vi "Run_Init Core.vi"(0 "functionbase in":refnum<class "functionbase.lvclass">, 11 "error in (no error)":errorcluster) -> (4 "functionbase out":refnum<class "functionbase.lvclass">, 15 "error out":errorcluster)   [LabVIEW 2019, in "LSL.lvlib" / "functionbase.lvclass"]
uses:
  functionbase.lvclass
  functionbase.lvclass/functionbase.ctl
  properties/Read Func Full String.vi
  properties/Read RT Variables.vi
  variables/RT Variables/RT Variables.lvclass
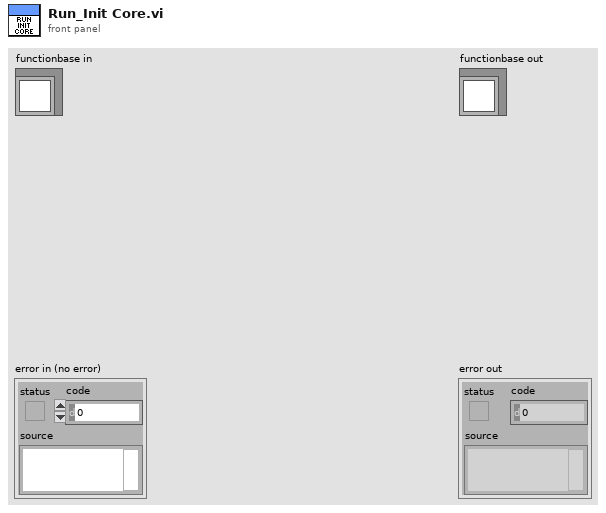
[diagram p1: front panel]
types:
  T1 = typedef "Datatype.ctl" = enum16{"Null", "Numeric", "String", "Bool", "Numeric 1D", "String 1D", "Bool 1D", "Numeric 2D", "String 2D", "Bool 2D", "Variant"}
  T2 = typedef "Valuetype.ctl" = enum16{"Value", "Variable", "Function"}
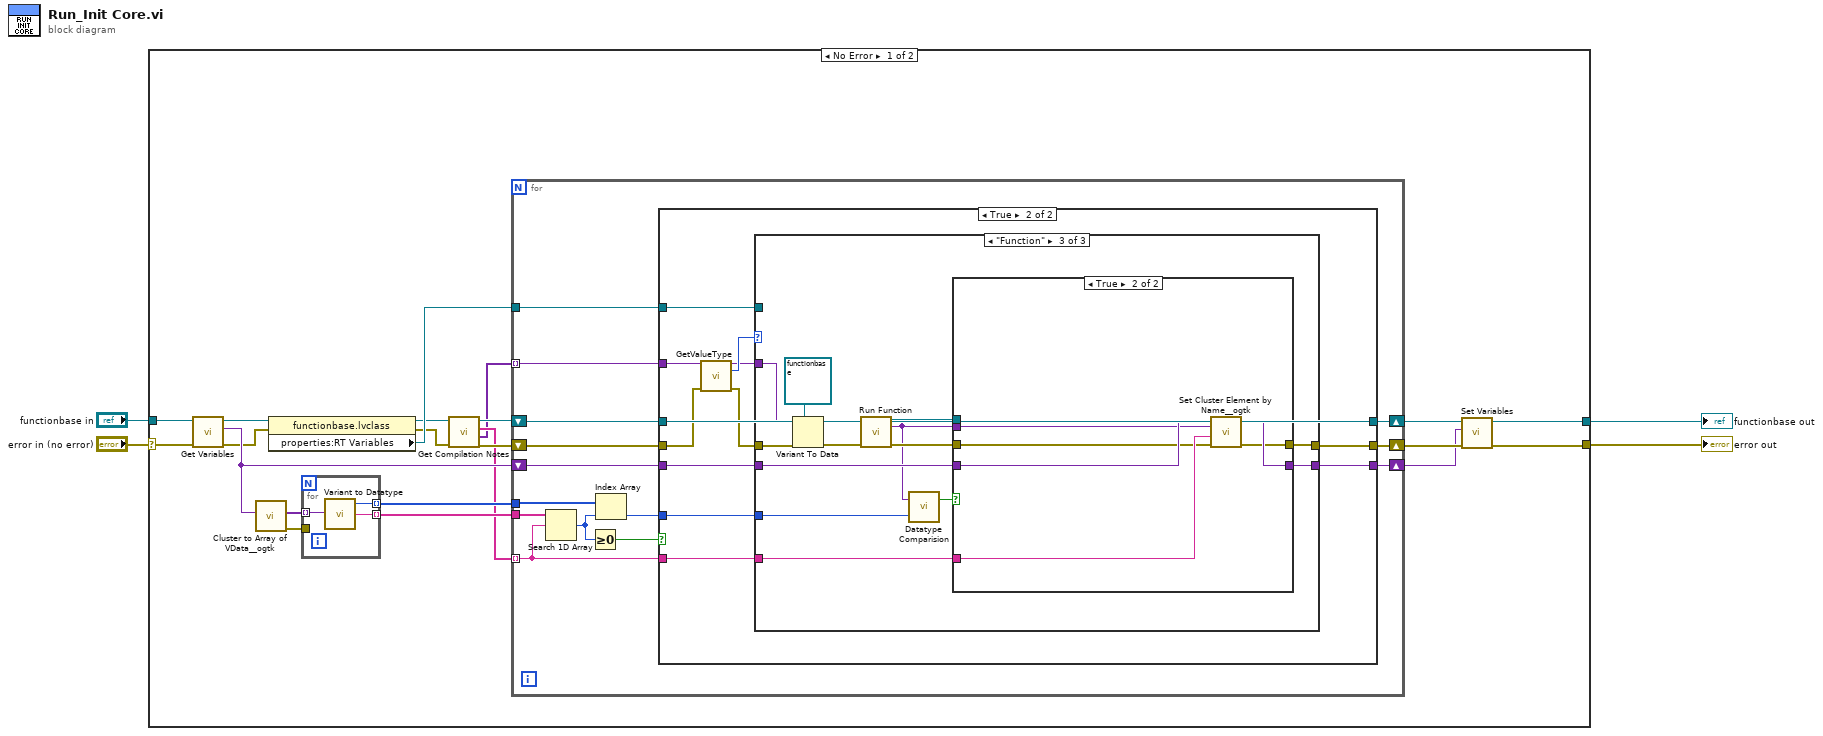
[diagram p0: block diagram]
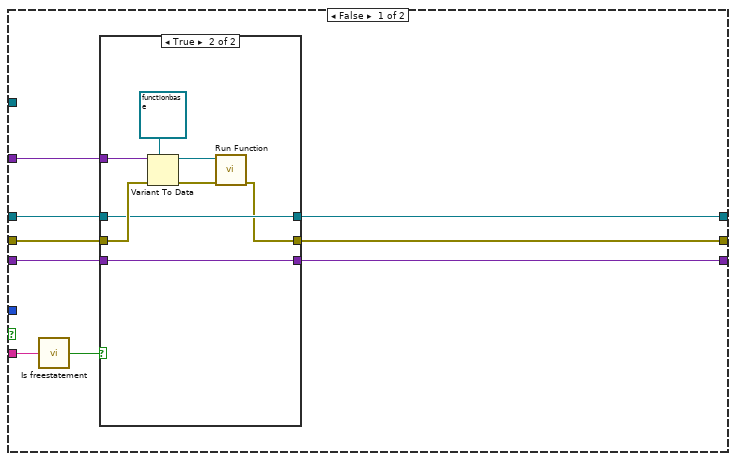
[diagram p2: hidden frame]
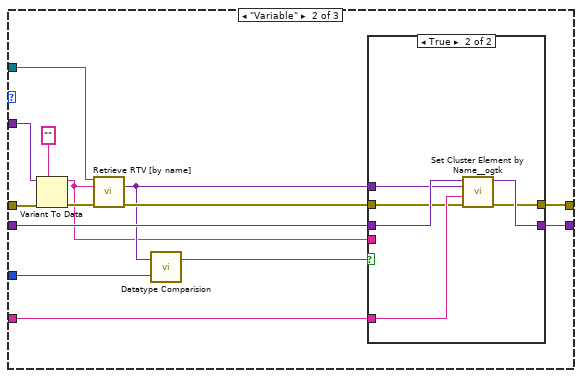
[diagram p5: hidden frame]
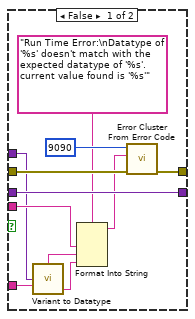
[diagram p6: hidden frame]
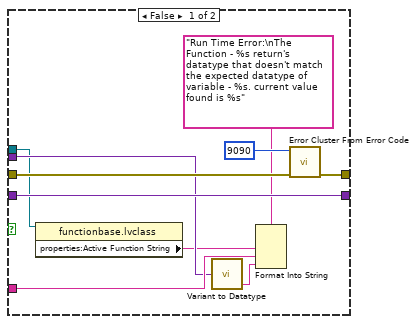
[diagram p7: hidden frame]
diagram:
  n1 = case shown="No Error" "error in (no error)" {
    selector: "error in (no error)" -> [w24 w138]
    tunnel: [w16 w138] -> w3
    tunnel: [w15 w137] -> w1
    tunnel: "functionbase in" -> [w23 w137]
    frame No Error {
      n2 = call-dynamic "Get Variables.vi"("error in (no error)"=w24, "functionbase in"=w23) -> ("error out"=w12:errorcluster, "Variables"=w20:variant, "functionbase out"=w13:refnum<class "functionbase.lvclass">)  [unwired: 7 in]
      n3 = call <userlib>:"Cluster to Array of VData__ogtk.vi"("Cluster"=w20) -> ("error out"=w22:errorcluster, "Array of VData"=w25:variant[])  [unwired: 9 in]
      n4 = property class="functionbase.lvclass"(reference=w13, error in=w12) -> (reference out=w10:refnum<class "functionbase.lvclass">, error out=w7:errorcluster, "properties:RT Variables"=w11:refnum<class "RT Variables.lvclass">)
      n5 = for {
        tunnel: w25 -> [w136] mode=indexing
        tunnel: [w135] -> w14 mode=indexing
        tunnel: [w134] -> w21 mode=indexing
        tunnel: w22 -> [_]
        n6 = call "Variant to Datatype.vi"("Variant"=w136) -> ("Name"=w134:string, "Datatype"=w135:T1)  [unwired: 2 in, 1 out]
      }
      n7 = call "Get Compilation Notes.vi"("error in (no error)"=w7, "functionbase in"=w10) -> ("error out"=w8:errorcluster, "note"=w5:variant[], "note Key"=w6:string[], "functionbase out"=w9:refnum<class "functionbase.lvclass">)  [unwired: 6 in]
      n8 = for {
        shift-right: [w36] -> w19
        shift-left: w9 -> [w34]
        tunnel: w21 -> [w32]
        shift-right: [w38] -> w17
        shift-left: w20 -> [w39]
        shift-right: [w37] -> w18
        shift-left: w8 -> [w33]
        tunnel: w14 -> [w31]
        tunnel: w11 -> [w35]
        tunnel: w6 -> [w26] mode=indexing
        tunnel: w5 -> [w27] mode=indexing
        n9 = Search 1D Array(1D array=w32, element=w26) -> (index of element=w30:i32)  [unwired: 1 in]
        n10 = Greater Or Equal To 0?(x=w30) -> (x >= 0?=w29:bool)
        n11 = Index Array(array=w31, index=w30) -> (element=w28:T1)
        n12 = case shown="True" w29 {
          tunnel: w39 -> [w41 w65]
          tunnel: [w42 w66] -> w38
          tunnel: w34 -> [w43 w71]
          tunnel: w33 -> [w46 w69]
          tunnel: w27 -> [w40 w70]
          tunnel: [w45 w64] -> w37
          tunnel: [w44 w71] -> w36
          tunnel: w28 -> [_ w62]
          tunnel: w26 -> [w48 w61]
          tunnel: w35 -> [_ w60]
          frame False {
            n13 = call "Is freestatement.vi"("Variable Name"=w48) -> ("freestatement?"=w47:bool)
            n14 = case shown="True" w47 {
              tunnel: w46 -> [w51 w56]
              tunnel: [w51 w53] -> w45
              tunnel: [w50 w55] -> w44
              tunnel: w43 -> [w50 w55]
              tunnel: [w49 w52] -> w42
              tunnel: w41 -> [w49 w52]
              tunnel: w40 -> [_ w54]
              frame False {
              }
              frame True {
                n15 = Variant To Data(error in=w56, type=refnum<class "functionbase.lvclass"> refnum ("functionbase.lvclass"), Variant=w54) -> (data=w57:refnum<class "functionbase.lvclass">, error out=w58:errorcluster)
                n16 = call-dynamic "Run Function.vi"("functionbase in"=w57, "error in (no error)"=w58) -> ("error out"=w53:errorcluster)  [unwired: 11 in, 2 out]
              }
            }
          }
          frame True {
            n17 = call "GetValueType.vi"("variant"=w70, "error in"=w69) -> ("variant out"=w67:variant, "Value Type"=w68:T2, "error out"=w63:errorcluster)  [unwired: 11 in]
            n18 = case shown="\"Function\"" w68 {
              tunnel: w67 -> [_ w86 w116]
              tunnel: [w73 w82 w112] -> w66
              tunnel: w65 -> [w73 w83 w113]
              tunnel: [w72 w81 w109] -> w64
              tunnel: w63 -> [w72 w87 w117]
              tunnel: w62 -> [_ w78 w107]
              tunnel: w61 -> [_ w79 w111]
              tunnel: w60 -> [_ w76 _]
              frame "Value", Default {
              }
              frame "Variable" {
                n19 = Variant To Data(error in=w87, type="", Variant=w86) -> (data=w74:string, error out=w84:errorcluster)
                n20 = call-dynamic "Retrieve RTV [by name].vi"("RT Variables in"=w76, "RTV name"=w74, "error in (no error)"=w84) -> ("Data"=w75:variant, "error out"=w80:errorcluster)  [unwired: 8 in, 3 out]
                n21 = call "Datatype Comparision.vi"("Required Datatype"=w78, "Data"=w75) -> ("Equal?"=w77:bool)  [unwired: 1 out]
                n22 = case shown="True" w77 {
                  tunnel: w83 -> [w97 w103]
                  tunnel: [w97 w102] -> w82
                  tunnel: w75 -> [w89 w101]
                  tunnel: w79 -> [w90 w100]
                  tunnel: w80 -> [w96 w99]
                  tunnel: [w95 w98] -> w81
                  tunnel: w74 -> [w91 _]
                  frame False {
                    n23 = call "Variant to Datatype.vi"("Variant"=w89) -> ("Value"=w88:string)  [unwired: 2 in, 2 out]
                    n24 = Format Into String(format string="Run Time Error:\nDatatype of '%s' doesn't match with the expected datatype of '%s'. current value found is '%s'" ("error message (\"\")"), w91, w90, w88) -> (resulting string=w92:string)  [unwired: 2 in, 1 out]
                    n25 = call <vilib>:"Error Cluster From Error Code.vi"("error in (no error)"=w96, "error message (\"\")"=w92, "error code (0)"=9090) -> ("error out"=w95:errorcluster)  [unwired: 6 in]
                  }
                  frame True {
                    n26 = call <userlib>:"Set Cluster Element by Name__ogtk.vi"("error in (no error)"=w99, "Element Name (\"\": New Element Data Name)"=w100, "New Element Value"=w101, "Cluster"=w103) -> ("error out"=w98:errorcluster, "VCluster out"=w102:variant)  [unwired: 5 in, 1 out]
                  }
                }
              }
              frame "Function" {
                n27 = Variant To Data(error in=w117, type=refnum<class "functionbase.lvclass"> refnum ("functionbase.lvclass"), Variant=w116) -> (data=w105:refnum<class "functionbase.lvclass">, error out=w114:errorcluster)
                n28 = call-dynamic "Run Function.vi"("functionbase in"=w105, "error in (no error)"=w114) -> ("functionbase out"=w104:refnum<class "functionbase.lvclass">, "Return"=w108:variant, "error out"=w110:errorcluster)  [unwired: 11 in]
                n29 = call "Datatype Comparision.vi"("Required Datatype"=w107, "Data"=w108) -> ("Equal?"=w106:bool)  [unwired: 1 out]
                n30 = case shown="True" w106 {
                  tunnel: w113 -> [w127 w133]
                  tunnel: [w127 w132] -> w112
                  tunnel: w108 -> [w120 w131]
                  tunnel: w111 -> [w121 w130]
                  tunnel: w110 -> [w126 w129]
                  tunnel: [w125 w128] -> w109
                  tunnel: w104 -> [w119 _]
                  frame False {
                    n31 = property class="functionbase.lvclass"(reference=w119) -> ("properties:Active Function String"=w118:string)  [unwired: 1 in, 2 out]
                    n32 = call "Variant to Datatype.vi"("Variant"=w120) -> ("Value"=w123:string)  [unwired: 2 in, 2 out]
                    n33 = Format Into String(format string="Run Time Error:\nThe Function - %s return's datatype that doesn't match the expected datatype of variable - %s. current value found is %s" ("error message (\"\")"), w118, w121, w123) -> ()  [unwired: 2 in, 2 out]
                    n34 = call <vilib>:"Error Cluster From Error Code.vi"("error in (no error)"=w126, "error code (0)"=9090) -> ("error out"=w125:errorcluster)  [unwired: 7 in]
                  }
                  frame True {
                    n35 = call <userlib>:"Set Cluster Element by Name__ogtk.vi"("error in (no error)"=w129, "Element Name (\"\": New Element Data Name)"=w130, "New Element Value"=w131, "Cluster"=w133) -> ("error out"=w128:errorcluster, "VCluster out"=w132:variant)  [unwired: 5 in, 1 out]
                  }
                }
              }
            }
          }
        }
      }
      n36 = call-dynamic "Set Variables.vi"("error in (no error)"=w18, "Variables"=w17, "functionbase in"=w19) -> ("error out"=w16:errorcluster, "functionbase out"=w15:refnum<class "functionbase.lvclass">)  [unwired: 7 in]
    }
    frame Error {
    }
  }
  "error out" <- w3
  "functionbase out" <- w1
